vi "UHR-Fleezers Control (host) - 10.5.vi"() -> ()   [LabVIEW 2011] (continued)
  in  "AI2 to Setpoint":cluster{"Set 1":bool, "Set 2":bool}
  out "AI2 (V)":cluster{"Set 1":dbl, "Set 2":dbl}={"Set 1"=0.008545182653279214, "Set 2"=0.00793481246375927}
  in  "Reset Feedback":cluster{"Set 1":bool, "Set 2":bool}
  in  "PID Gains":T9={"Set 1"={"proportional gain (Kc)"=0, "integral gain (Kc*Ts/Ti)"=5, "derivative gain (Kc*Td/Ts)"=0}, "Set 2"={"proportional gain (Kc)"=0, "integral gain (Kc*Ts/Ti)"=5, "derivative gain (Kc*Td/Ts)"=0}}
  in  "Feedback On/Off":cluster{"Set 1":bool, "Set 2":bool}={"Set 1"=TRUE, "Set 2"=TRUE}
  in  "Rem fb disp offset":bool caption="Rem. Offset"
  in  "Remove Unwinding Offset":bool
  in  "FB Trap Pos Offset":dbl=-0.7109037245680824 caption="Offset (nm)" format="%.1f"
  in  "Negate Y Axis":bool=TRUE
  in  "Set Reading to\nSetpoint":bool
  out "Trap X (AI1)":T10={"Trap 1"=-0.21429443359375, "Trap 2"=-0.115386962890625}
  in  "Trap Pos FB SP":fxp<+/-,16,1>=-0.099884033203125 caption="Setpoint"
  in  "Trap Pos. FB ON":bool
  in  "Reset Trap Pos. FB":bool
  out "Trap Positions":waveform(dbl)[](graph)=[{"t0"=timestamp(16.200000000000017 s since 1904-01-01), "dt"=0.15, "Y"=[-0.7109037245680824, -0.7109037245680824], "attributes"=variant("NI_ChannelName"=variant(string "Trap 1 Pos."))}, {"t0"=timestamp(16.200000000000017 s since 1904-01-01), "dt"=0.15, "Y"=[-6.991740519879386e-12, -6.991740519879386e-12], "attributes"=variant("NI_ChannelName"=variant(string "Trap 2 Pos."))}]
  in  "Tab Control 8":enum32{"Main Setting", "Details"}(tab)=enum."Details"
  in  "Trap Pos FB Int Count":u16=100
  in  "Trap Pos. FB Gains":T11={"proportional gain (Kc)"=10.0, "integral gain (Kc*Ts/Ti)"=10.0, "derivative gain (Kc*Td/Ts)"=0.0} {"proportional gain (Kc)" format="%.11g"; "integral gain (Kc*Ts/Ti)" format="%.11g"; "derivative gain (Kc*Td/Ts)" format="%.11g"}
  in  "Negate Diff?":bool=TRUE
  in  "Differential FB?":bool=TRUE
  in  "Trap Pos. FB Offset Factor":i64
  in  "Trap Pos FB Negate Action":bool
  in  "Trap Pos. FB Mult Factor":i64=16777216
  in  "Trap Pos. AI1 X Pre-scale":u16
  in  "Trap Pos. FB Range":T12={"output high"=0.999969482421875, "output low"=-1.0}
  out "Trap Pos FB Int Signal":fxp<+/-,24,9>=0.0328369140625 format="%.18g"
  out "Trap Pos FB Int-Norm Signal":fxp<+/-,16,1>=0.000335693359375 format="%.16g"
  in  "Set SP Using...":bool
  in  "Trap Pos FB Monitor\nT1 or T2":bool
  out "Trap X AI1 (DMA)":T13={"Set 1"=-0.192901611328125, "Set 2"=-0.203460693359375}
  in  "N El. to Ave.":dbl=10000.0
  out "Trap Pos FB Action":i64
  out "Action (%)":dbl(knob) scale=-100.0..100.0
  in  "Trap Pos. FB Out Scale 2^n":u8=24 caption="Action Scale Factor"
  out "Mean T1 Position (nm)":dbl=-0.7109037245680824 caption="Mean T1 (nm)" format="%0.2f"
  out "Trap 1 Position RMS (A)":dbl caption="RMS (Ang)"
  in  "Remove Action Offset":bool
  in  "factor":dbl=0.8
  in  "Trap Pos. Disp. Downsample":dbl=10000.0 caption="Trap Downsample"
  in  "Tab Control 3":enum32{"Timing", "MCL Scan", "Analog Out"}(tab)
  out "APD 2 Gate Late Counter":u32
  out "APD 2 Gate Relative Phase":i16
  in  "Phase Adj. (APD 2 Gate)":i16=20
  in  "Initial Phase Adjustment (APD 2 Gate)":i16=55
  out "APD 1 Gate Late Counter":u32
  in  "- phase (APD 1 Gate)":bool
  in  "+ phase (APD 1 Gate)":bool
  out "APD 1 Gate Relative Phase":i16
  in  "Phase Adj. (APD 1 Gate)":i16=20
  in  "Initial Phase Adjustment (APD 1 Gate)":i16=60
  in  "Save APD Data\nwith Trap Data":bool=TRUE
  out "APD FIFO Elements Remaining":u32
  in  "- phase (APD Acq)":bool
  in  "+ phase (APD Acq)":bool
  out "APD Acq Late Counter":u32
  out "APD Acq Relative Phase":i16
  in  "Phase Adj. (APD Acq)":i16=20
  in  "Initial Phase Adjustment (APD Acq)":i16
  in  "Invert APD Gate":bool caption="Invert Gate"
  in  "APD Gate OFF Count":u32=450 caption="Gate OFF Count"
  in  "APD Gate ON Count":u32=150 caption="Gate ON Count"
  in  "APD Gate":enum32{"ON", "OFF", "Interlace"}(radio)=enum."Interlace"
  in  "APD Integration Time (s)":dbl=0.01 caption="Integration Time (s)"
  out "APD Acq Rate (Hz)":dbl=100.0 caption="Rate (Hz)"
  out "APD Samples/FIFO Acq.":dbl=30.0
  out "APD Elements/DMA read":u32=60
  out "APD Int. Count":u32=400000 format="%.0p"
  in  "+ phase (APD 2 Gate)":bool
  in  "- phase (APD 2 Gate)":bool
  in  "Tab Control 5":enum32{"PSD X", "PSD Y", "Other Data Channel"}(tab)
  out "Data map":dbl[][](graph)=[[0.021232040412682448, 0.029264234925337584, 0.029006221486001793, 0.02947332252742222, 0.08117035353983584, 0.08125846758312531, 0.08158726536152129, 0.08103929314907515, 0.08086431250910761, 0.08095055673850357, 0.0810326053804941, 0.08121217706602767, 0.08130585875437957, 0.08119153979287855, 0.0807736066773429, 0.0808730065805841, 0.08034219289721328, 0.08065756573352731, 0.0798441911191358, 0.08064908607469315], [0.02154942255276071, 0.029251847737439093, 0.02928519395399211, 0.029671065228562832, 0.08098177014562143, 0.08112784968736758, 0.0818703356211826, 0.0819009773022203, 0.08153339157143549, 0.08141921248731046, 0.08125436154206075, 0.08198482377612497, 0.08141641046869738, 0.08147861034542062, 0.08110951316345694, 0.08080458286142964, 0.08065619157642165, 0.08036829380570791, 0.08070979430427827, 0.08033721827780646], [0.021170968901117932, 0.02945360907754016, 0.029276257052076052, 0.029432007951534563, 0.0814690252904354, 0.08205679006691108, 0.08281121861781308, 0.0829614261664322, 0.08349217019996226, 0.0831732431297363, 0.08326838013859794, 0.0831837885705323, 0.08335734804632525, 0.08206119257594857, 0.08153556534178173, 0.08139490483961481, 0.0810984156367747, 0.08067855104420052, 0.08034314390893962, 0.08047188539951261], [0.02164561110399326, 0.029430226935626635, 0.0296883570243495, 0.02999846906012186, 0.08363320795606122, 0.08465743100576079, 0.08593018166876956, 0.08674696824361813, 0.0876337878737849, 0.08730915089207796, 0.08759303412245067, 0.08646169072556753, 0.08583766702898205, 0.08460134431579552, 0.08301847393778736, 0.08216762380860021, 0.0816487455157143, 0.08139314206493467, 0.08046417791955601, 0.08063321329911374], [0.021104812530504915, 0.02994358682992274, 0.03038731094412813, 0.03157360704090748, 0.0873264618986491, 0.08871967968125948, 0.09041132278732258, 0.09241431971546124, 0.09310078169290839, 0.09279532396576136, 0.09264218058510947, 0.09188700798917543, 0.09031297124465333, 0.08756408512507073, 0.08575282765772123, 0.08415796302654197, 0.0827430249012936, 0.08189603181725667, 0.08079185549052113, 0.08143078809750585], [0.0223851606274997, 0.030857562411567483, 0.03224400591013252, 0.033915634174343734, 0.09079507413002623, 0.09256727602984466, 0.09476373353453094, 0.0961825663712632, 0.09649550359107258, 0.09642431879678381, 0.09589758114604388, 0.09551232632910817, 0.09385614698374493, 0.09073141176026817, 0.0881665346370158, 0.08608034798429662, 0.08378809608563498, 0.08217425646759832, 0.08130132008407012, 0.08105820944807904], [0.023022934242175615, 0.03181609689489803, 0.03390003252442557, 0.03558078336711946, 0.09130062164396671, 0.09291239667404705, 0.09446113061726638, 0.09495307857345867, 0.0949683425320649, 0.0944176751195131, 0.09433456560417214, 0.094512418466156, 0.09362225865518572, 0.09169877502578228, 0.08932386699666928, 0.08700364650937732, 0.0846298351458831, 0.08242456987827512, 0.08141262443406477, 0.081253727166313], [0.023486119536245326, 0.032028619484785435, 0.03342976461288319, 0.03523875188238414, 0.08882689446376614, 0.0895076903046651, 0.08944936153386293, 0.09031435828264972, 0.09000099996316324, 0.08944442516286026, 0.0894052639635168, 0.08998322637270048, 0.0900060635988309, 0.08861502879979855, 0.0874994013404857, 0.0856407362789437, 0.083897310471859, 0.08194663032092604, 0.0814385941007056, 0.08101698163579069], [0.022779453577030283, 0.031098622510979973, 0.031730739716791634, 0.03297951202940194, 0.0848578278212771, 0.08493454548820525, 0.08482584802759702, 0.08466877188219246, 0.08451197369977337, 0.08462732333119766, 0.08378009583145937, 0.08454233792944607, 0.08415838652011993, 0.08416446809975459, 0.08353734667940621, 0.08245855871569575, 0.08166186612115992, 0.08116188542346575, 0.08082852647738746, 0.08111938368935528], [0.022330269630825027, 0.029401507544873584, 0.029537826365148144, 0.030093889917130745, 0.08047610785248974, 0.08006415639480492, 0.08046952112373394, 0.08040455598518687, 0.08026529632246968, 0.0796075772707935, 0.07956118720773958, 0.08007991067377232, 0.07915336539067325, 0.07887896914056709, 0.07867305190506818, 0.0794425834332329, 0.07924141929098552, 0.0791598333354738, 0.07979954901526429, 0.07977330818564615], [0.02044033449076586, 0.028130984672381513, 0.027366236953036534, 0.02736498348795648, 0.0764467834442511, 0.07638850849593458, 0.07626170751351175, 0.07618015618034456, 0.07604688081977751, 0.07548223058564817, 0.07476740908149276, 0.0744830280359572, 0.07441787046677945, 0.07420936275560092, 0.07525632220417226, 0.0761120899709385, 0.07760392883850695, 0.07844515486333616, 0.07870717446153982, 0.07908199465387289], [0.019942869953335204, 0.026763260441673653, 0.0255163747934697, 0.024952581713883693, 0.07292787014378843, 0.07216618925984775, 0.0721656450513236, 0.07121732690403365, 0.07032424641995136, 0.07037858759908261, 0.0699806895119518, 0.06944926660882329, 0.0695489822862552, 0.0708572779591253, 0.07223823474485636, 0.07404510557794941, 0.07618809909966273, 0.07745869912088685, 0.0788160997396248, 0.07937980411590129], [0.020475159507784016, 0.026401365259331594, 0.025125151020287093, 0.023628366063837017, 0.07147388366488497, 0.06946304171014732, 0.06904634772138057, 0.06764585362271133, 0.06699246640120121, 0.06650691187589554, 0.06635540364977774, 0.06674964952328469, 0.06756152437130694, 0.06952383440191429, 0.07190062943944654, 0.07455435469596067, 0.07657428012584738, 0.07797323694898181, 0.07869591733130829, 0.07933393584745521], [0.020726229865859744, 0.02687344433091808, 0.025495753170754802, 0.02417315626935109, 0.07243533512691333, 0.06989073371829398, 0.06864676696716483, 0.06751665334276241, 0.06669750663277076, 0.06615143076047911, 0.06693786553650335, 0.06774990796820946, 0.0695168424149924, 0.0712350869623194, 0.07366794766772458, 0.07562024749671925, 0.07736534436136949, 0.07877477142598321, 0.07953786218297608, 0.07993831027799944], [0.021558173271615307, 0.02752309762438901, 0.026646455640265188, 0.025438660388374335, 0.07511021096373065, 0.07316701605981638, 0.0719915705042528, 0.07071014524521022, 0.07038208928349671, 0.07008114987426783, 0.0702495351443466, 0.07129785627477556, 0.07245228001850479, 0.07429506648876733, 0.07622488075268116, 0.0781263675154797, 0.07883258530654616, 0.07931246378917903, 0.07946737358748221, 0.07972169216918507], [0.02194399522887953, 0.027797536227585552, 0.027137530297039067, 0.027343628325165355, 0.07744516234613569, 0.07645612950213976, 0.07595436962345298, 0.07512038615364845, 0.0750719994201199, 0.07482729081663736, 0.07508902844836403, 0.0758669470679669, 0.07628483360806061, 0.0775562559097139, 0.07843623369771069, 0.0796982080324068, 0.07985300531124397, 0.07971351569336307, 0.08000108337025785, 0.08009265428808329], [0.021742493698836712, 0.028255237209208053, 0.02807463484647008, 0.027920757852026315, 0.07870911506058714, 0.07831055764863733, 0.07820031376681036, 0.07793146494114082, 0.07800798054111158, 0.07803182969026103, 0.07790154344099817, 0.07818214160237774, 0.07864912558010435, 0.07887135080059629, 0.07948676103090543, 0.07967259636918395, 0.08010516965244695, 0.08072767918514245, 0.08028216355134932, 0.0806830552805923], [0.0214291763767935, 0.028081221215855566, 0.02783161008094924, 0.02828810229680509, 0.07939499461314559, 0.0792176405299245, 0.07855017398576203, 0.07903344798118872, 0.0785780922795315, 0.07876615613199647, 0.07910967598384405, 0.07875921993301523, 0.07962041667478997, 0.07970039037848733, 0.07954399133752615, 0.08008848881149032, 0.08042816571669616, 0.08027799072338784, 0.08002265668829543, 0.08058001195360057], [0.021907175885851685, 0.027842220897654438, 0.028006974299907166, 0.028316076434475437, 0.07962024488187, 0.07886435507008427, 0.07901798260395251, 0.0787343105713231, 0.07921665782680276, 0.07902075748228872, 0.07918818753659262, 0.07880512709912212, 0.0799199074420031, 0.07992987283644706, 0.07987365311074514, 0.08019600894419922, 0.08073735821823519, 0.08019179933425621, 0.08005922753457435, 0.08001284684609242], [0.022031768161914912, 0.027312396642023496, 0.02819203644821005, 0.02850026423269944, 0.07915208659105216, 0.07917303429190647, 0.07916166794337309, 0.07936572868585814, 0.07898664834804611, 0.07938680799623066, 0.07904743307028719, 0.07948319031546291, 0.07997892142574847, 0.07997173080613044, 0.08080009317157719, 0.07985320917659236, 0.0802461461779197, 0.08029811365482746, 0.07993008535196533, 0.0807440715957421], [0.02167386981766506, 0.027634000667122162, 0.028169027060627176, 0.028917155616581446, 0.07961258409981625, 0.07918354201221985, 0.07951881878530334, 0.0795397766699425, 0.07945286629648274, 0.0797050012331013, 0.07935858027012124, 0.07995815472042522, 0.0800854139112942, 0.08044112734420043, 0.08055582466836317, 0.08019910227285199, 0.07991218799210333, 0.08009558094515284, 0.0794524341149438, 0.0806167360810302], [0.02184732421900258, 0.028292149832369384, 0.028254629135782833, 0.02846383825732109, 0.08004798290280425, 0.07983852612317618, 0.07972584320776283, 0.07939153125355565, 0.07965965002667119, 0.0799284591108816, 0.08025920320520198, 0.07991869094808426, 0.08011112590984842, 0.08062228896977029, 0.08038581871439587, 0.07979218553899578, 0.08051923559640084, 0.08039819511929022, 0.07987820829970399, 0.08010737366361806], [0.021945183194045974, 0.028316327650740682, 0.028333405955279133, 0.028597599099288717, 0.0801914333850135, 0.08002157591302458, 0.0797951833140822, 0.08017325830116241, 0.07971599770459281, 0.08006531848004979, 0.08016300028224169, 0.08009865611310282, 0.08024238745154674, 0.08064456664868092, 0.08035267850984898, 0.08021273090218689, 0.08074112115393092, 0.08033040554921608, 0.08015554081339345, 0.07997002023867383], [0.022013208603734555, 0.028073978258364572, 0.028531395115721656, 0.02903341948772981, 0.08044528756103803, 0.08021552118948003, 0.07997337235029015, 0.08021153971645059, 0.08018934758514581, 0.08025120107672913, 0.08044731136968797, 0.08014741082482939, 0.08001962958667683, 0.08039371794058092, 0.08026659192987691, 0.08010684144500521, 0.08025403928627697, 0.08059948446368337, 0.07995995030673353, 0.0801262359996369], [0.021952340608445815, 0.02792459599185297, 0.029214125274435093, 0.029702009013707217, 0.08020547330488449, 0.07954191904345656, 0.07962561161116524, 0.07978248430808348, 0.07977811303692416, 0.08019904715873039, 0.08007660068643371, 0.08021864822112655, 0.07978964035341453, 0.08005661348314674, 0.08027173373126312, 0.08012250610472374, 0.08021940331967672, 0.08014791616626495, 0.08005899785321646, 0.08014845059283426], [0.021581230398775943, 0.02817111408797794, 0.029222450703307354, 0.029958536508221417, 0.08011010732633694, 0.07959231118701221, 0.07957138990939855, 0.07938826217438694, 0.07936290398033408, 0.0799600037244977, 0.0799403059181194, 0.08012312227926507, 0.0796978413186925, 0.08000627971493683, 0.0801547129845677, 0.08020875385182882, 0.08019970755884774, 0.07965064847007475, 0.07980201634169615, 0.08042164510834096], [0.021799687545018376, 0.027843496058511816, 0.02895678956210647, 0.04829985338180308, 0.07956187638892073, 0.07972928982764034, 0.07986739013137636, 0.07969893790790919, 0.07946776916387482, 0.08000780536071325, 0.07958583751274925, 0.07993884794597084, 0.07957239185955044, 0.07945475013343958, 0.07998597888282372, 0.08011513488522794, 0.07996290013565496, 0.07948359752502258, 0.08054526224014501, 0.07977591856922217], [0.021670863322083296, 0.02783788769140987, 0.02857791500134089, 0.05469628966247977, 0.0797161576995428, 0.07954428616834489, 0.07985814809773636, 0.08015250233153015, 0.07986918881863002, 0.08024813081889726, 0.0797883626265046, 0.08014410758023999, 0.08019494903342309, 0.07953955426584156, 0.0803913851323783, 0.08045961512268851, 0.079859028578294, 0.08010174498193988, 0.08048756388339867, 0.08012282815931837], [0.0219680761536891, 0.026118578071360553, 0.02822125739653116, 0.05403934659439866, 0.07960237423556177, 0.07954166953736551, 0.08003667973047748, 0.08004041448139795, 0.07996061438141157, 0.08009609915609436, 0.08002544695860625, 0.08027026102628115, 0.0803660992841737, 0.07990183547736561, 0.08038906705026852, 0.08016734928059069, 0.08005506789293973, 0.07983874349843681, 0.08029028392293691, 0.08024899001938088], [0.021506620787658443, 0.02613200743783909, 0.027914043680207522, 0.05354246380036743, 0.07998990527312122, 0.08010579153504252, 0.08010334122234408, 0.07982070197379545, 0.08026681781928241, 0.07990945958558054, 0.08016765901368746, 0.08051544685568023, 0.07992350581090638, 0.08028116307320092, 0.07983329717360715, 0.08014029438273523, 0.07974404484312261, 0.08025144655995335, 0.08023172959296909, 0.08038420419368031], [0.02126554301280267, 0.02614178650490209, 0.027799533886148125, 0.05349654961034766, 0.08027111491789743, 0.07986746166482958, 0.08050518598481263, 0.07989855953389971, 0.08040114483468488, 0.0800799798345532, 0.08024854686896218, 0.08073629017685521, 0.0803121812225664, 0.08096976803488733, 0.08046966866252574, 0.0803159494166393, 0.08005501799046888, 0.07995939495688884, 0.08016286551456264, 0.07987427862920453], [0.021530529123318473, 0.026235810246569395, 0.027966440490109427, 0.053680111761135386, 0.08065916397239331, 0.08012089180300216, 0.0802086441553132, 0.08076027078111017, 0.08050942686731849, 0.08017190574698407, 0.08068245093776394, 0.08050236389594378, 0.08036803077549023, 0.08070071808705491, 0.08074795495100687, 0.08030108389844781, 0.07983318350511728, 0.0798875499546311, 0.0802048533450547, 0.08063171817941034], [0.021516256078642007, 0.02619650948103422, 0.028243259693354568, 0.05418968547938244, 0.08031344681819769, 0.08050053177377431, 0.07999316299823095, 0.08067699418707931, 0.08070727894227724, 0.08036948079131181, 0.08048247071813056, 0.08074383026098314, 0.08088759468765713, 0.08058731630711324, 0.0804135504941918, 0.08024062937562716, 0.08042044158432383, 0.08038826431368025, 0.08033360034084913, 0.08025571072431861], [0.021651495679137357, 0.026158850605783074, 0.028283345383060016, 0.05457664279342314, 0.08013496952053492, 0.08037643809127498, 0.07997734684233115, 0.08047465907356083, 0.08024388212578501, 0.08045073641871739, 0.08040769600805878, 0.08093282084475126, 0.08059737498992087, 0.08073786123001042, 0.08056136362728243, 0.08007860928602648, 0.080533450018733, 0.07997882975128814, 0.0799969968302876, 0.0805479661473195], [0.02189741008104431, 0.0264896784251652, 0.028486276085346703, 0.05460809594361807, 0.08028843281504633, 0.08036867234345761, 0.08017194980750078, 0.08078881310491313, 0.08087588937942145, 0.08061393519982746, 0.08036487415806282, 0.080655287301307, 0.080415767801861, 0.08030284531604953, 0.08054850176321189, 0.0802852691641468, 0.08015318607624211, 0.08014691064624913, 0.08030961818629023, 0.08017703009023011], [0.021452942512913305, 0.027177048580048196, 0.028361880866891568, 0.054262808664831186, 0.08041478312126951, 0.08065669732110248, 0.0803026315109433, 0.08054848301402831, 0.08079180770250685, 0.0802432601728128, 0.08023336271939277, 0.08063941902375812, 0.08109486723988343, 0.08042426984171885, 0.0804959791061867, 0.08093951734601953, 0.08033611967223386, 0.08020085085002815, 0.08028577358528896, 0.08065086331063079], [0.021056713663731887, 0.027358593706871007, 0.02837893028712409, 0.05449278751393874, 0.08050691790272321, 0.0809209420228719, 0.0803493585611743, 0.08099095122378598, 0.08050947452672805, 0.080575036226576, 0.08029079845158696, 0.08053120206504569, 0.08069728275999463, 0.08118328960359228, 0.08023730541730209, 0.0803544242799144, 0.07998159710348313, 0.08061266919218107, 0.08021496885920795, 0.080429505121484], [0.020859421460156503, 0.02655241304769932, 0.028338427339950643, 0.0542953583303642, 0.08064803148830975, 0.08013495822265426, 0.08009407347178936, 0.08032752059014736, 0.080376539834487, 0.08044891925834609, 0.08060410301769919, 0.08065085691802971, 0.08063771109077475, 0.08055982321578647, 0.08098194306349876, 0.08061908507869199, 0.0799339396450914, 0.08048776279635361, 0.08000927323261067, 0.0807316048166163], [0.021088775919887566, 0.02554844331827863, 0.028303421141457112, 0.054589357473087546, 0.0803622219012473, 0.08012204176363302, 0.08024770422791964, 0.08003935648213312, 0.08023654178679522, 0.08066299033714186, 0.08078237167498555, 0.08058330653326805, 0.0808269374636429, 0.08089301378211589, 0.08088577832899185, 0.08059412301735305, 0.08015327046763371, 0.0803271225432857, 0.08001237438360194, 0.08060477767592619], [0.021506120206039932, 0.025488927170924165, 0.02832099730192697, 0.05466636726804954, 0.08048404072930143, 0.08036940482264818, 0.08004529369122548, 0.08036674431752314, 0.08062680608998159, 0.08062376238924446, 0.08072200549142237, 0.08047312511575597, 0.08112310051907123, 0.0806290590178948, 0.08022894908236704, 0.0797370872513239, 0.07998367085620517, 0.08028440068059839, 0.08031986821243998, 0.08029038251619416]]
  in  "Channel":i32=4
  in  "Abort MCL Scan":bool
  out "MCL Scan I":u64
  out "MCL Scanning":bool
  in  "Start MCL Scan":bool
  out "wait to reset values":bool
  in  "Tab Control 4":enum32{"Scan Settings", "MCL FPGA Loop Timing"}(tab)
  out "Total Time (s)":dbl=48.0
  in  "Scan lines (y)":u64=20
  in  "Fast Scan Dir":bool=TRUE
  in  "2D or 1D Scan":bool=TRUE
  out "Initial X":dbl=-0.6096261482589191
  out "Initial Y":dbl=6.375612048707543
  out "Time/f+b scan (s) (MCL)":dbl=2.4 caption="Time/scan (s)"
  in  "Number of scans (MCL)":u64=1 caption="Scans"
  in  "Scan steps (MCL)":u64=40 caption="Scan steps (x)"
  in  "N APD Samp/step":dbl=3.0
  in  "Scan Range (V)\n(of steps)":dbl=3.5
  in  "Restart DMA? (MCL)":bool=TRUE caption="Restart DMA?"
  in  "Continuous MCL Scanning":bool caption="Cont. Scanning"
  in  "Center Scan":bool=TRUE
  in  "Save Data (MCL)":bool=TRUE caption="Save Data"
  out "Actual Incr. int (MCL)":i16=294 caption="Incr. int"
  out "Desired incr (int)":dbl=294.0628205128205
  out "Desired Scan Incr (V)":dbl=0.08974358974358974
  out "N sets should be saved (MCL)":dbl=160.0 caption="N sets should be saved"
  out "Data points/scans (MCL)":dbl=4800.0 caption="Data points/scans"
  out "Data points/scan (f+b)":dbl=240.0 caption="points/scan (f+b)"
  out "Cycles/step (MCL)":u64=2000 caption="Cycles/step" format="%.0p"
  out "Actual MCL Inc (V)":dbl=0.08972441785943175
  in  "Phase adjust (MCL)":i16 caption="Phase adjust"
  out "Relative Phase (MCL)":i16 caption="Relative Phase"
  in  "Initial Phase Adj. (MCL)":i16 caption="Initial Phase Adj."
  in  "Update Count (MCL)":u32=600
  in  "+ phase (MCL)":bool
  in  "- phase (MCL)":bool
  out "MCL Late Counter":u32
  in  "APD 1 AO Mult.":i16=1 min=1
  in  "APD 2 AO Mult.":i16=1 min=1
  in  "Tab Control 7":enum32{"Green FB Signals", "Slow MCL Scan"}(tab)
  out "Green FB Plot":dbl(graph)=0.08941923276467177
  out "MCL Scan 2":cluster{"Begin (V)":dbl, dbl, dbl[]}(graph)
  out "MCL Scan":cluster{"Begin (V)":dbl, dbl, dbl[]}(graph)
  in  "Green laser mode":enum32{"Laser ON", "Laser OFF", "Interlace"}(radio)=enum."Interlace"
  in  "GI Frequency, ON count":u32=150 min=1 step=1
  in  "Invert GI":bool
  out "GI Late Counter":u32
  in  "Phase adj. (GI)":i16=5
  out "GI relative phase":i16
  in  "+ phase (GI)":bool
  in  "Initial Phase Adjustment (GI)":i16=19
  in  "GI Frequency, OFF count":u32=450 min=1 step=1
  in  "- phase (GI)":bool
  out "Green FB Signals (V)":cluster{"Y":dbl, "X":dbl, "Sum":dbl}={"Y"=111.83276450511946, "X"=111.83276450511946, "Sum"=0.08941923276467177}
  out "Relative phase (Green FB)":i16
  in  "+ phase (Green FB)":bool
  in  "- phase (Green FB)":bool
  out "Green FB Count":u32=600
  in  "Phase adj. (Green FB)":i16=10
  in  "Initial Phase Adjustment (Green FB)":i16=50
  in  "Green FB On/Off":bool=TRUE
  in  "Current When FB OFF (%)":dbl=87.0 min=0.0 max=100.0 step=1.0
  in  "Green int current ON count adj":u32=150
  in  "Green FB Gains":T14={"proportional gain (Kc)"=10, "integral gain (Kc*Ts/Ti)"=5, "derivative gain (Kc*Td/Ts)"=0}
  in  "- phase (GI) 2":bool
  in  "Initial Phase Adjustment (GI) 2":i16=-100
  in  "+ phase (GI) 2":bool
  out "GI relative phase 2":i16
  in  "Phase adj. (GI) 2":i16=20
  out "GI Late Counter 2":u32
  in  "On one out of X cycles":u32=1
  in  "Trap Position FIFO Depth":u32=300000 format="%.0p"
  in  "# Samples/trap":u32=20000 format="%.0p"
  out "Trap AI Elements/DMA read":u32=320000 format="%.0p"
  out "Ave. Rate (Hz)":dbl=200000.0 format="%#_6p"
  out "FIFO El. Rem.":u32 format="%.0p"
  in  "Phase adj. (AI1)":i16=15
  out "Relative phase (AI1)":i16
  in  "+ phase (AI1)":bool
  in  "- phase (AI1)":bool
  out "Late Counter (AI1)":u32
  in  "Initial Phase Adjustment (AI1)":i16=220
  out "AI rate (Hz)":dbl=200000.0 format="%#_6p"
  in  "AI Count (ticks)":u32=200
  out "# Samples/channel":u32=40000 format="%.0p"
  in  "Trap AI FIFO Depth":u32=600000 format="%.0p"
  in  "Detector Type":string(combo)="IR-QPD + PSD + FB-QPD X position"
